vi "Process Temporary View Layers.vi"(5 "Delete Selected Area?":bool, 6 "Valid Selection?":bool, 7 "Data in":T1={"Class"={"Ants"=refnum, "Layer"=refnum, "Templates"=refnum, "Icon"=refnum, "Glyph"=refnum, "Settings"=refnum, "Tools"=refnum}, "Ref"={"Add Layer"=refnum, "Remove Layer"=refnum, "Line Text"=[], "Body Text Spec"=refnum, "DNL_Font"=refnum, "glyph path str"=refnum, "templates path str"=refnum, "Arrow Up"=refnum, "Arrow Down"=refnum, "IE VI Ref"=refnum, "Glyphs tree"=refnum, "Templates tree"=refnum, "Layer Icon Text"=refnum, "Layer Template"=refnum, "Body Text"=refnum, "Search Templates"=refnum, "TextMarker"=refnum, "Tab Control"=refnum, "Search Glyphs"=refnum, "Line Color"=refnum, "DNL_Glyphs []"=refnum, "Fill Color"=refnum, "Tools"=refnum, "Icon"=refnum, "Preview"=refnum, "Ants"=refnum, "Terminals"=refnum, "menu reference"=refnum, "LayerNames"=[], "GlyphLoadAnimation"=refnum, "TemplateLoadAnimation"=refnum, "refreshGlyphs"=refnum, "refreshTemplates"=refnum}, "Support"={"AntsRect"={"left"=0, "top"=0, "right"=0, "bottom"=0}, "Mouse Move Coords"={"Horizontal"=0, "Vertical"=0}, "Mouse Down Coords"={"Horizontal"=0, "Vertical"=0}, "Temp Coord"={"Horizontal"=0, "Vertical"=0}, "Action"=enum."Default", "Edge Color"=4914962, "Fill Color"=16860, "Mouse Down?"=FALSE, "Draft Mode?"=FALSE, "Temp Icon"=bytes[3102], "CTRL Pressed"=FALSE, "Move Selection?"=FALSE, "AntsRect Orig"={"left"=0, "top"=0, "right"=0, "bottom"=0}, "Text"="", "TM Set?"=FALSE, "Mouse inside icon?"=FALSE, "Tool (old value)"=0, "Pencil Move Color"=0, "Swap Colors?"=FALSE, "Shift pressed?"=FALSE}}, 8 "error in (no error)":errorcluster, 9 "Layer Locked?":bool, 10 "#Active Layer":i32, 11 "All Layers in":refnum<class "Layer.lvclass">[](array[class])) -> (0 "error out":errorcluster, 2 "Locked?":bool, 3 "All Layers out":refnum<class "Layer.lvclass">[](array[class]))   [LabVIEW 2021]
uses:
  <vilib>/LabVIEW Icon API/lv_icon/Classes/Layer/Layer.lvclass
  <resource>/plugins/NIIconEditor/Controls/Global Data.ctl
  <resource>/plugins/NIIconEditor/Class/Ants/Ants.lvclass
  <resource>/plugins/NIIconEditor/Class/FakedArray/FakedArray.lvclass
  <vilib>/LabVIEW Icon API/lv_icon/Classes/Icon/Icon.lvclass
  <resource>/plugins/NIIconEditor/Class/Icon Library/Glyph.lvclass
  <resource>/plugins/NIIconEditor/Class/Settings/Settings.lvclass
  <resource>/plugins/NIIconEditor/Class/Tools/Tools Paint.lvclass
  <resource>/plugins/NIIconEditor/Controls/IE Classes.ctl
  <resource>/plugins/NIIconEditor/Controls/References Cluster.ctl
  <resource>/plugins/NIIconEditor/Controls/SupportClass.ctl
  <vilib>/Utility/miscctls.llb/LVPoint32TypeDef.ctl
  <resource>/plugins/NIIconEditor/Controls/SupportClass_Action.ctl
  <vilib>/LabVIEW Icon API/lv_icon/Controls/IEColor.ctl
  <vilib>/LabVIEW Icon API/lv_icon/Controls/Layer.ctl
  <vilib>/LabVIEW Icon API/lv_icon/lv_icon.lvlib
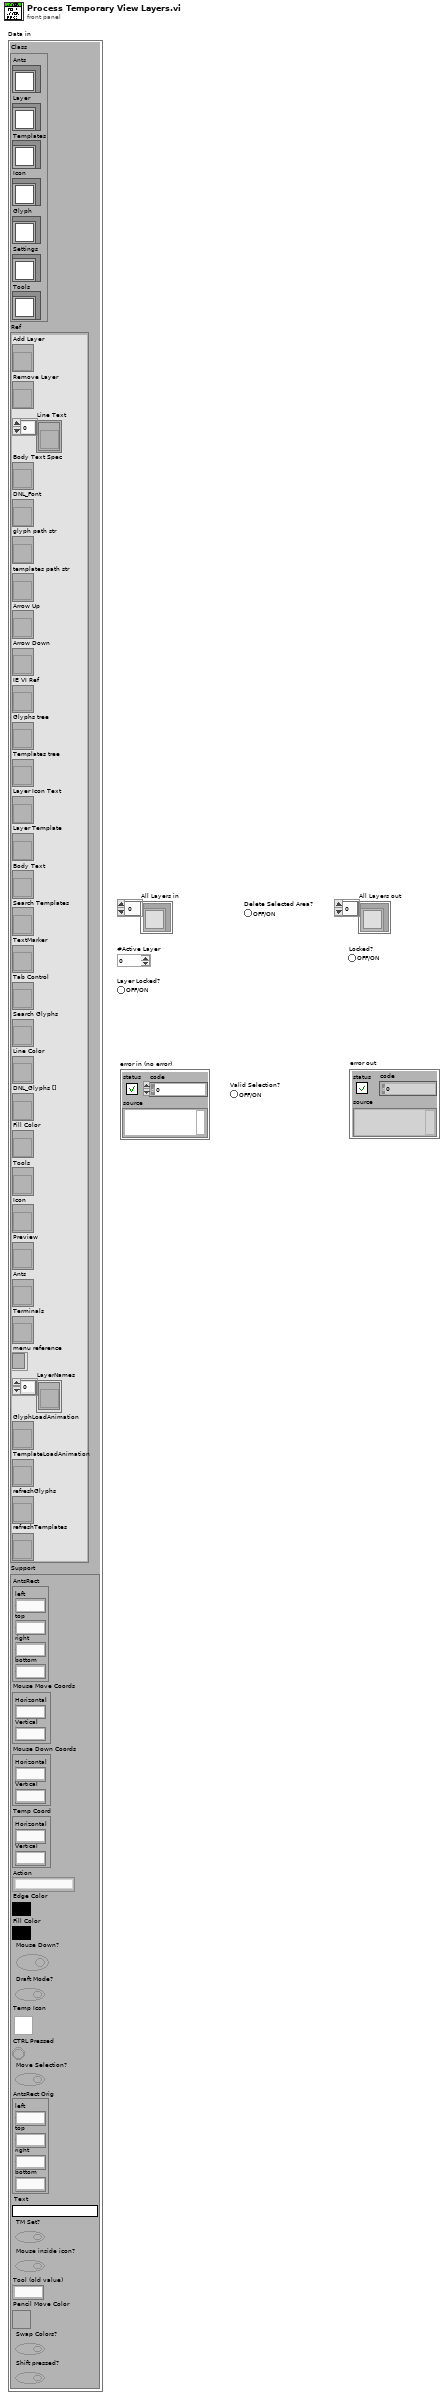
[diagram p1: front panel]
types:
  T1 = typedef "lv_icon.lvlib/Global Data.ctl" = cluster{"Class":T2, "Ref":T3, "Support":T4}
  T2 = typedef "IE Classes.ctl" = cluster{"Ants":refnum<class "Ants.lvclass">, "Layer":refnum<class "FakedArray.lvclass">, "Templates":refnum<class "FakedArray.lvclass">, "Icon":refnum<class "Icon.lvclass">, "Glyph":refnum<class "Glyph.lvclass">, "Settings":refnum<class "Settings.lvclass">, "Tools":refnum<class "Tools Paint.lvclass">}
  T3 = typedef "lv_icon.lvlib/References Cluster.ctl" = cluster{"Add Layer":refnum<vi>, "Remove Layer":refnum<vi>, "Line Text":refnum<vi>[], "Body Text Spec":refnum<vi>, "DNL_Font":refnum<vi>, "glyph path str":refnum<vi>, "templates path str":refnum<vi>, "Arrow Up":refnum<vi>, "Arrow Down":refnum<vi>, "IE VI Ref":refnum<vi>, "Glyphs tree":refnum<vi>, "Templates tree":refnum<vi>, "Layer Icon Text":refnum<vi>, "Layer Template":refnum<vi>, "Body Text":refnum<vi>, "Search Templates":refnum<vi>, "TextMarker":refnum<vi>, "Tab Control":refnum<vi>, "Search Glyphs":refnum<vi>, "Line Color":refnum<vi>, "DNL_Glyphs []":refnum<vi>, "Fill Color":refnum<vi>, "Tools":refnum<vi>, "Icon":refnum<vi>, "Preview":refnum<vi>, "Ants":refnum<vi>, "Terminals":refnum<vi>, "menu reference":refnum<k9>, "LayerNames":refnum<vi>[], "GlyphLoadAnimation":refnum<vi>, "TemplateLoadAnimation":refnum<vi>, "refreshGlyphs":refnum<vi>, "refreshTemplates":refnum<vi>}
  T4 = typedef "SupportClass.ctl" = cluster{"AntsRect":cluster{"left":i16, "top":i16, "right":i16, "bottom":i16}, "Mouse Move Coords":T5, "Mouse Down Coords":T5, "Temp Coord":T5, "Action":T6, "Edge Color":T7, "Fill Color":T7, "Mouse Down?":bool, "Draft Mode?":bool, "Temp Icon":picture, "CTRL Pressed":bool, "Move Selection?":bool, "AntsRect Orig":cluster{"left":i16, "top":i16, "right":i16, "bottom":i16}, "Text":string, "TM Set?":bool, "Mouse inside icon?":bool, "Tool (old value)":u32, "Pencil Move Color":u32, "Swap Colors?":bool, "Shift pressed?":bool}
  T5 = typedef "LVPoint32TypeDef.ctl" = cluster{"Horizontal":i32, "Vertical":i32}
  T6 = typedef "SupportClass_Action.ctl" = enum16{"Default", "Move Selection", "Glyph Library", "Tool"}
  T7 = typedef "IEColor.ctl" = u32
  T8 = cluster{"left":i16, "top":i16, "right":i16, "bottom":i16}
  T9 = cluster{"left":i32, "top":i32, "right":i32, "bottom":i32}
  T10 = typedef "Layer.ctl" = cluster{"LayerIcon":picture, "LayerName":string, "Opacity":u8, "Visibility?":bool}
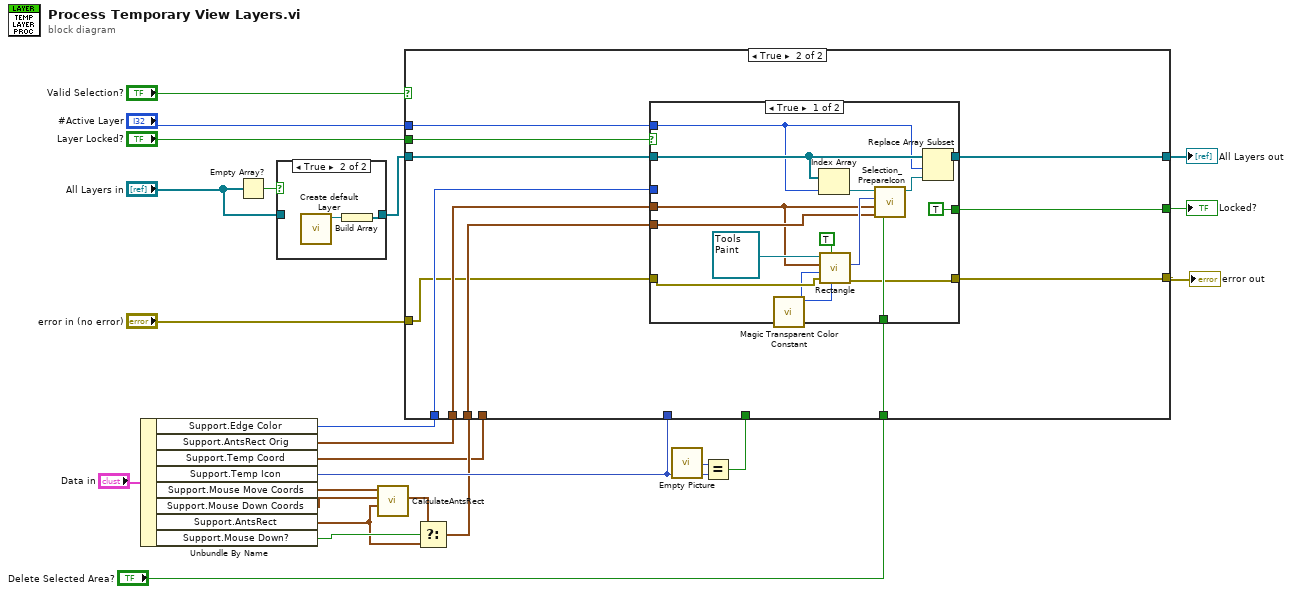
[diagram p0: block diagram]
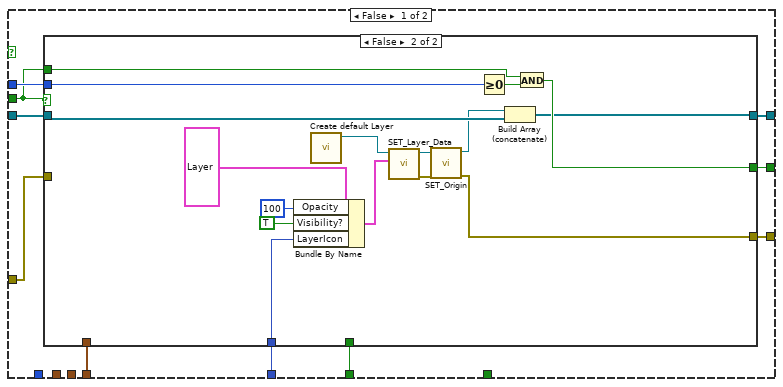
[diagram p2: hidden frame]
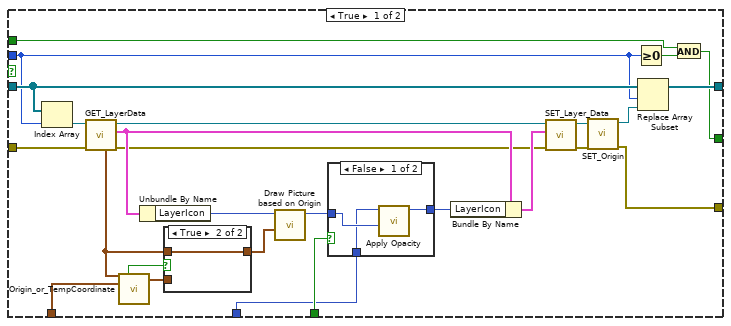
[diagram p3: hidden frame]
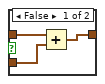
[diagram p4: hidden frame]
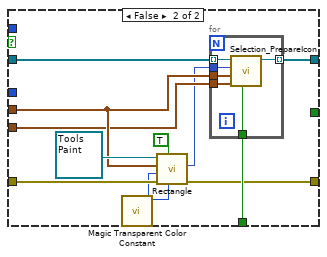
[diagram p6: hidden frame]
diagram:
  n1 = Unbundle By Name("Data in") -> ("Support.Edge Color"=w11:T7, "Support.AntsRect Orig"=w12:T8, "Support.Temp Coord"=w13:T5, "Support.Temp Icon"=w24:picture, "Support.Mouse Move Coords"=w16:T5, "Support.Mouse Down Coords"=w17:T5, "Support.AntsRect"=w20:T8, "Support.Mouse Down?"=w21:bool)
  n2 = Empty Array?(array="All Layers in") -> (empty?=w10:bool)
  n3 = case shown="True" w10 {
    tunnel: [w25 w27] -> w8
    tunnel: "All Layers in" -> [w25 _]
    frame False {
    }
    frame True {
      n4 = call <vilib>:"Create default Layer.vi"() -> ("Layer.lvclass out"=w26:refnum<class "Layer.lvclass">)  [unwired: 1 in, 10 out]
      n5 = Build Array(w26) -> (w27:refnum<class "Layer.lvclass">[])
    }
  }
  n6 = call <resource>:"CalculateAntsRect.vi"("AntsRect"=w20, "Mouse Down Coords"=w17, "Mouse Move Coords"=w16) -> ("Rect"=w14:cluster{i32, i32, i32, i32})  [unwired: 8 out]
  n7 = Select(t=w14, s=w21, f=w20) -> (s? t:f=w15:T9)
  n8 = call "Empty Picture"() -> ("empty picture"=w22:picture)
  n9 = Equal?(x=w22, y=w24) -> (x = y?=w23:bool)
  n10 = case shown="True" "Valid Selection?" {
    tunnel: w13 -> [w37 _]
    tunnel: [w36 w92] -> w9
    tunnel: w8 -> [w35 w97]
    tunnel: "#Active Layer" -> [w34 w96]
    tunnel: [w33 w91] -> w6
    tunnel: "Layer Locked?" -> [w28 w98]
    tunnel: w15 -> [_ w94]
    tunnel: w12 -> [_ w95]
    tunnel: w11 -> [_ w93]
    tunnel: "Delete Selected Area?" -> [_ w90]
    tunnel: w23 -> [w32 _]
    tunnel: w24 -> [w31 _]
    tunnel: "error in (no error)" -> [w30 w89]
    tunnel: [w29 w88] -> w2
    frame False {
      n11 = case shown="False" w28 {
        tunnel: w37 -> [w63 _]
        tunnel: [w62 w79] -> w36
        tunnel: w35 -> [w61 w78]
        tunnel: w34 -> [w60 w87]
        tunnel: [w59 w86] -> w33
        tunnel: w32 -> [w45 _]
        tunnel: w28 -> [w44 w82]
        tunnel: w31 -> [w43 w75]
        tunnel: w30 -> [w42 _]
        tunnel: [w40 w80] -> w29
        frame True {
          n12 = Index Array(array=w61, index=w60) -> (element=w55:refnum<class "Layer.lvclass">)
          n13 = call-dynamic "GET_LayerData.vi"("error in (no error)"=w42, "Layer.lvclass in"=w55) -> ("error out"=w38:errorcluster, "Data"=w58:T10, "Layer.lvclass out"=w54:refnum<class "Layer.lvclass">, "Origin"=w56:T5)  [unwired: 6 out]
          n14 = call <resource>:"Origin_or_TempCoordinate.vi"("Origin"=w56, "Temp Coord"=w63) -> ("Temp?"=w47:bool, "Origin out"=w57:T5)  [unwired: 24 out]
          n15 = Unbundle By Name(w58) -> ("LayerIcon"=w52:picture)
          n16 = case shown="True" w47 {
            tunnel: w56 -> [w66 w67]
            tunnel: w57 -> [w65 _]
            tunnel: [w64 w67] -> w50
            frame False {
              n17 = Add(x=w66, y=w65) -> (x+y=w64:T5)
            }
            frame True {
            }
          }
          n18 = call <vilib>:"Draw Picture based on Origin.vi"("Origin"=w50, "LayerIcon in"=w52) -> ("LayerIcon out"=w39:picture)  [unwired: 1 in, 8 out]
          n19 = case shown="False" w45 {
            tunnel: [w70 w71] -> w51
            tunnel: w43 -> [w68 _]
            tunnel: w39 -> [w69 w71]
            frame False {
              n20 = call <vilib>:"Apply Opacity.vi"("Bottom"=w69, "Top"=w68) -> ("new picture"=w70:picture)  [unwired: 1 in, 8 out]
            }
            frame True {
            }
          }
          n21 = Bundle By Name(cluster=w58, "LayerIcon"=w51) -> (w53:T10)
          n22 = call-dynamic "SET_Layer_Data.vi"("error in (no error)"=w38, "Data"=w53, "Layer.lvclass in"=w54) -> ("error out"=w41:errorcluster, "Layer.lvclass out"=w48:refnum<class "Layer.lvclass">)  [unwired: 1 in, 6 out]
          n23 = call-dynamic "SET_Origin.vi"("error in (no error)"=w41, "Layer.lvclass in"=w48) -> ("error out"=w40:errorcluster, "Layer.lvclass out"=w49:refnum<class "Layer.lvclass">)  [unwired: 1 in, 7 out]
          n24 = Greater Or Equal To 0?(x=w60) -> (x >= 0?=w46:bool)
          n25 = Replace Array Subset(array=w61, new element=w49, index=w60) -> (w62:refnum<class "Layer.lvclass">[])
          n26 = And(x=w44, y=w46) -> (x .and. y?=w59:bool)
        }
        frame False {
          n27 = Bundle By Name(cluster=T10 {"LayerIcon"=bytes[0], "LayerName"="", "Opacity"=0, "Visibility?"=FALSE} ("Data"), "Opacity"=u8 100, "Visibility?"=TRUE, "LayerIcon"=w75) -> (w85:T10)
          n28 = call <vilib>:"Create default Layer.vi"() -> ("Layer.lvclass out"=w74:refnum<class "Layer.lvclass">)  [unwired: 1 in, 10 out]
          n29 = call-dynamic "SET_Layer_Data.vi"("Data"=w85, "Layer.lvclass in"=w74) -> ("error out"=w81:errorcluster, "Layer.lvclass out"=w84:refnum<class "Layer.lvclass">)  [unwired: 2 in, 6 out]
          n30 = call-dynamic "SET_Origin.vi"("error in (no error)"=w81, "Layer.lvclass in"=w84) -> ("error out"=w80:errorcluster, "Layer.lvclass out"=w77:refnum<class "Layer.lvclass">)  [unwired: 1 in, 7 out]
          n31 = Greater Or Equal To 0?(x=w87) -> (x >= 0?=w83:bool)
          n32 = Build Array (concatenate)(w77, w78) -> (w79:refnum<class "Layer.lvclass">[])
          n33 = And(x=w82, y=w83) -> (x .and. y?=w86:bool)
        }
      }
    }
    frame True {
      n34 = case shown="True" w98 {
        tunnel: w97 -> [w112 w120]
        tunnel: w96 -> [w111 _]
        tunnel: w95 -> [w105 w123]
        tunnel: w94 -> [w106 w122]
        tunnel: w93 -> [_ _]
        tunnel: [w110 w119] -> w92
        tunnel: [TRUE _] -> w91
        tunnel: w90 -> [w103 w118]
        tunnel: w89 -> [w101 w116]
        tunnel: [w100 w115] -> w88
        frame True {
          n35 = call <vilib>:"Magic Transparent Color Constant.vi"() -> ("Magic transparent color constant"=w99:u32)  [unwired: 11 out]
          n36 = Index Array(array=w112, index=w111) -> (element=w108:refnum<class "Layer.lvclass">)
          n37 = call-dynamic "Rectangle.vi"("Fill Color"=w99, "fill?(F)"=TRUE, "error in (no error)"=w101, "Edge Color"=w99, "rect"=w105, "Tools Paint in"=refnum<class "Tools Paint.lvclass"> refnum) -> ("error out"=w100:errorcluster, "new picture"=w107:picture)  [unwired: 4 out]
          n38 = call <resource>:"Selection_PrepareIcon.vi"("Delete Selected Area?"=w103, "AntsRect"=w106, "AntsRect Orig"=w105, "new picture"=w107, "Layer.lvclass in"=w108) -> ("Layer.lvclass out"=w104:refnum<class "Layer.lvclass">)  [unwired: 6 out]
          n39 = Replace Array Subset(array=w112, new element=w104, index=w111) -> (w110:refnum<class "Layer.lvclass">[])
        }
        frame False {
          n40 = call <vilib>:"Magic Transparent Color Constant.vi"() -> ("Magic transparent color constant"=w114:u32)  [unwired: 11 out]
          n41 = call-dynamic "Rectangle.vi"("Fill Color"=w114, "fill?(F)"=TRUE, "error in (no error)"=w116, "Edge Color"=w114, "rect"=w123, "Tools Paint in"=refnum<class "Tools Paint.lvclass"> refnum) -> ("error out"=w115:errorcluster, "new picture"=w121:picture)  [unwired: 4 out]
          n42 = for {
            tunnel: w123 -> [w130]
            tunnel: w122 -> [w129]
            tunnel: w121 -> [w128]
            tunnel: w120 -> [w127] mode=indexing
            tunnel: [w126] -> w119 mode=indexing
            tunnel: w118 -> [w125]
            n43 = call <resource>:"Selection_PrepareIcon.vi"("Delete Selected Area?"=w125, "AntsRect"=w129, "AntsRect Orig"=w130, "new picture"=w128, "Layer.lvclass in"=w127) -> ("Layer.lvclass out"=w126:refnum<class "Layer.lvclass">)  [unwired: 6 out]
          }
        }
      }
    }
  }
  "All Layers out" <- w9
  "Locked?" <- w6
  "error out" <- w2
